vi "ArduinoRead.vi"(7 "Arduino function":enum16{"T/RH", "Interlock", "Edgesense"}(ring), 8 "error in (no error)":errorcluster, 9 "Humidity IN":dbl[](array[numeric]), 10 "Temperature IN":dbl[](array[numeric]), 11 "ArduinoControl in":refnum<class "ArduinoControl.lvclass">) -> (0 "error out":errorcluster, 1 "rel. Humidity [%]":dbl, 2 "Temperature [°C]":dbl, 3 "ArduinoControl out":refnum<class "ArduinoControl.lvclass">, 4 "Interlock Status":u16(ring) items=["Dark", "Light"], 5 "Edgesense Status":u16(ring)=1 items=["Contact", "No contact"])   [LabVIEW 2019, in "ArduinoControl.lvclass"]
uses:
  ArduinoControl.lvclass
  ArduinoControl.lvclass/ArduinoControl.ctl
panel:
  out "Humidity OUT":dbl[](array[numeric])
  out "Temperature OUT":dbl[](array[numeric])
  out "return count":u32
  out "String":string
  out "VISA resource name OUT":refnum<visa-resource-name>="COM24"
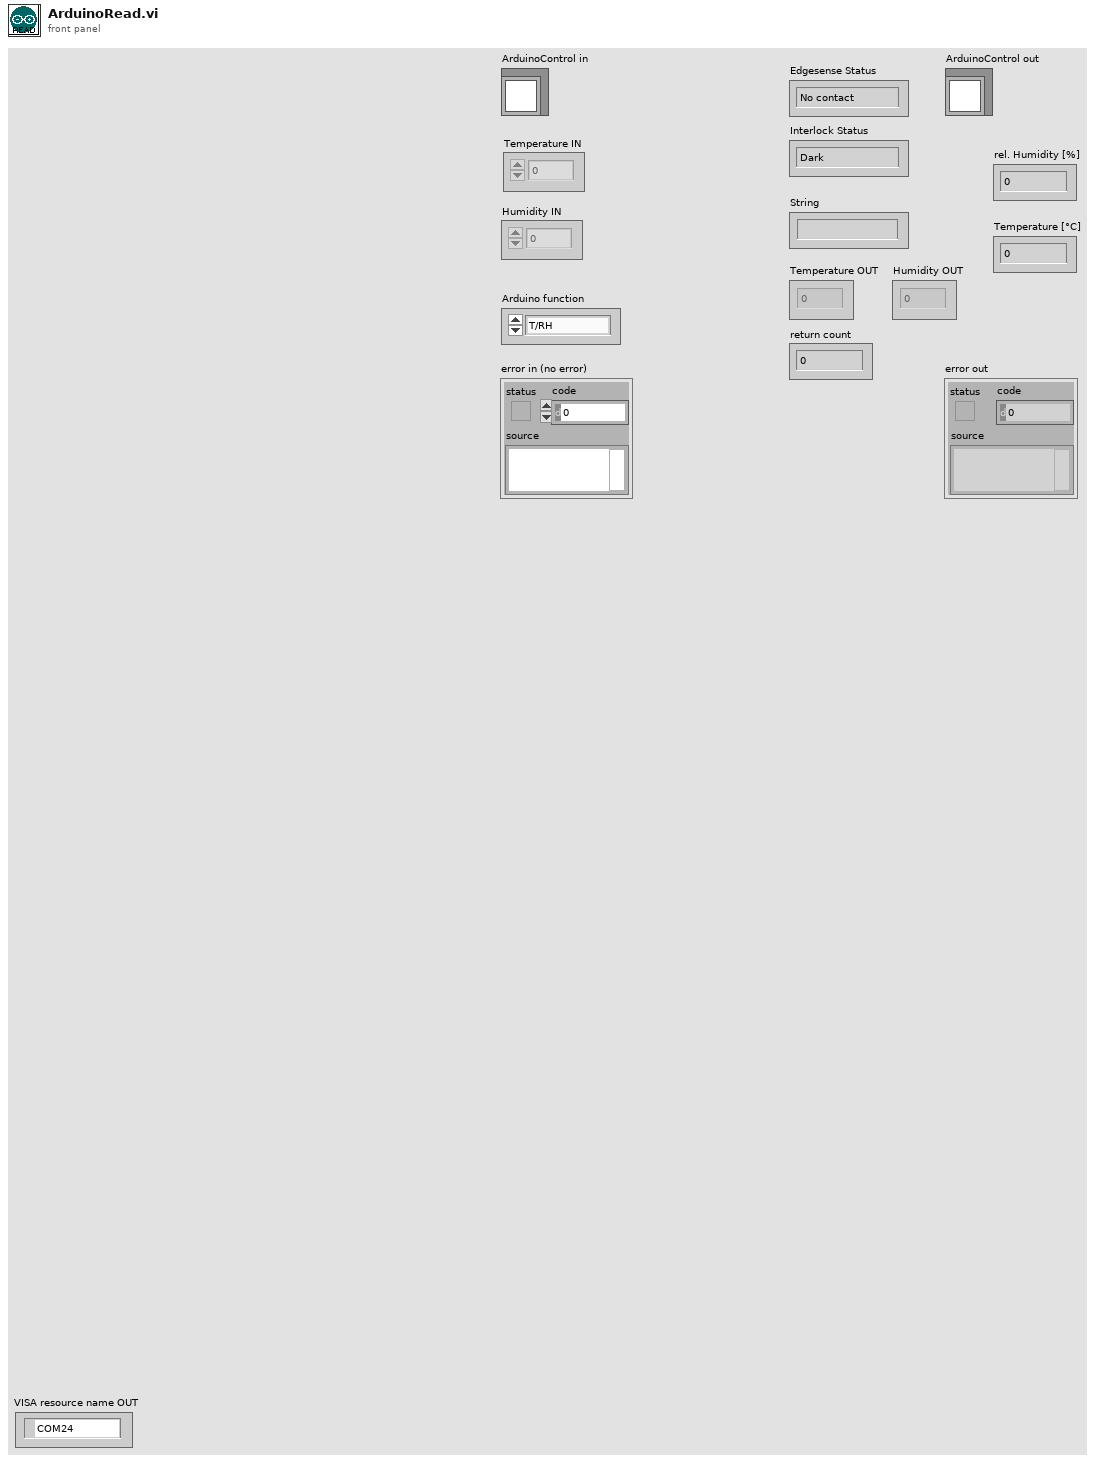
[diagram p1: front panel]
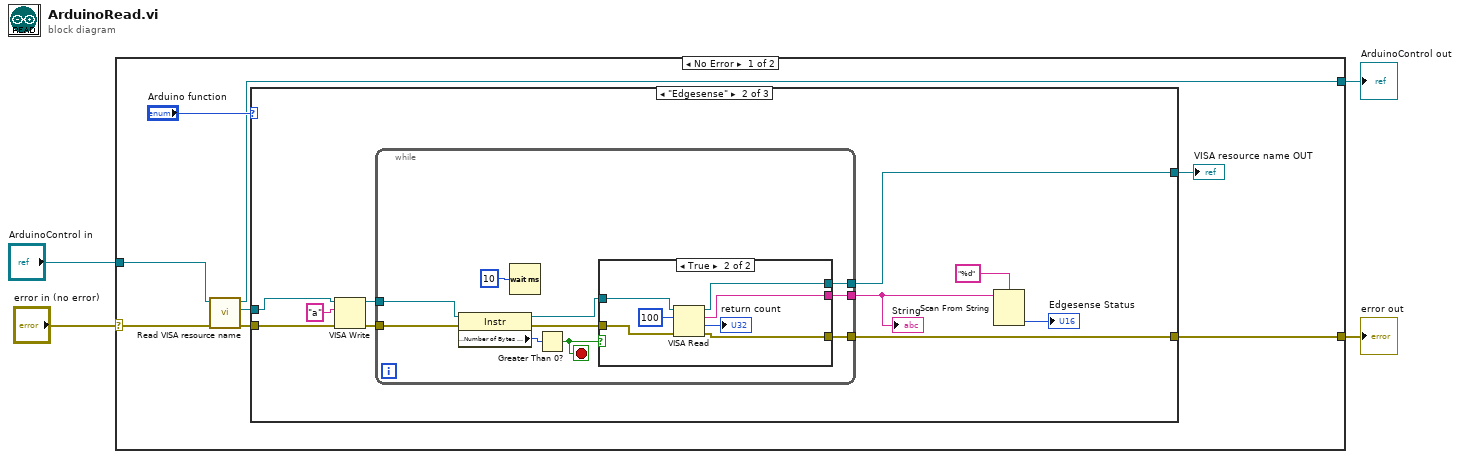
[diagram p0: block diagram]
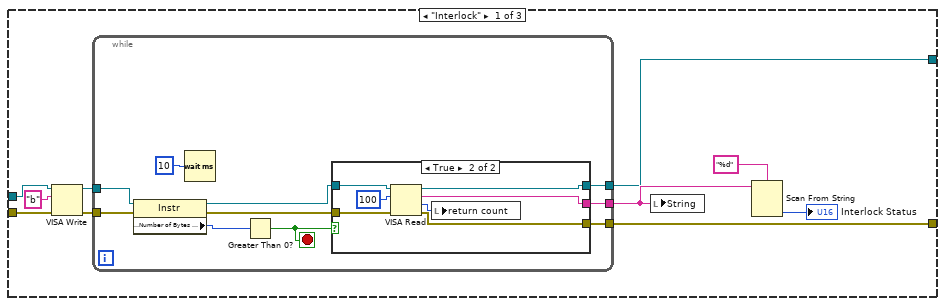
[diagram p2: hidden frame]
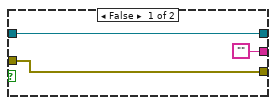
[diagram p3: hidden frame]
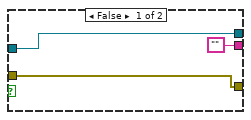
[diagram p4: hidden frame]
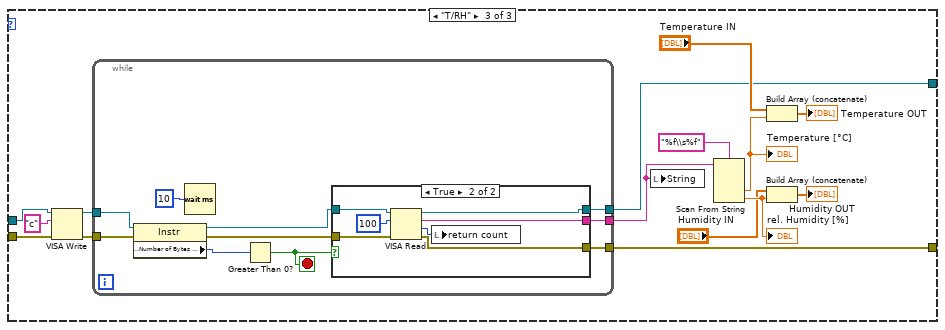
[diagram p5: hidden frame]
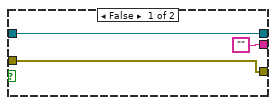
[diagram p6: hidden frame]
diagram:
  n1 = case shown="No Error" "error in (no error)" {
    selector: "error in (no error)" -> [w7 w109]
    tunnel: [w8 w108] -> w2
    tunnel: "ArduinoControl in" -> [w9 w108]
    tunnel: [w10 w109] -> w1
    frame No Error {
      n2 = call "Read VISA resource name.vi"("error in (no error)"=w7, "ArduinoControl in"=w9) -> ("error out"=w6:errorcluster, "VISA resource name"=w5:refnum<visa-resource-name>, "ArduinoControl out"=w8:refnum<class "ArduinoControl.lvclass">)  [unwired: 7 in]
      n3 = case shown="\"Edgesense\"" "Arduino function" {
        tunnel: w6 -> [w14 w45 w75]
        tunnel: w5 -> [w16 w46 w77]
        tunnel: [w19 w48 w78] -> w11
        tunnel: [w18 w49 w79] -> w10
        frame "Interlock" {
          n4 = VISA Write(VISA resource name=w16, write buffer="b", error in (no error)=w14) -> (VISA resource name out=w15:refnum<visa-resource-name>, error out=w13:errorcluster)  [unwired: 1 out]
          n5 = while {
            tunnel: [w30] -> w19
            tunnel: [w29] -> w20
            tunnel: w13 -> [w23]
            tunnel: w15 -> [w24]
            tunnel: [w28] -> w18
            stop <- w25 stop-if-true
            n6 = property class="Instr"(reference=w24, error in=w23) -> (reference out=w32:refnum<visa-resource-name>, error out=w31:errorcluster, "Serial Settings:Number of Bytes at Serial Port"=w26:u32)
            n7 = Wait (ms)(milliseconds to wait=10) -> ()  [unwired: 1 out]
            n8 = Greater Than 0?(x=w26) -> (x > 0?=w25:bool)
            n9 = case shown="True" w25 {
              tunnel: w32 -> [w33 w42]
              tunnel: w31 -> [w34 w41]
              tunnel: [w33 w40] -> w30
              tunnel: ["" w39] -> w29
              tunnel: [w34 w38] -> w28
              frame False {
              }
              frame True {
                n10 = VISA Read(VISA resource name=w42, byte count=100, error in (no error)=w41) -> (VISA resource name out=w40:refnum<visa-resource-name>, read buffer=w39:string, return count=w37:u32, error out=w38:errorcluster)
                n11 = local write "return count"(w37) -> ()
              }
            }
          }
          n12 = local write "String"(w20) -> ()
          n13 = Scan From String(format string="%d", input string=w20) -> (output 1=→"Interlock Status":u16)  [unwired: 3 in, 3 out]
        }
        frame "Edgesense" {
          n14 = VISA Write(VISA resource name=w46, write buffer="a", error in (no error)=w45) -> (VISA resource name out=w44:refnum<visa-resource-name>, error out=w43:errorcluster)  [unwired: 1 out]
          n15 = while {
            tunnel: [w60] -> w48
            tunnel: [w59] -> w50
            tunnel: w44 -> [w55]
            tunnel: [w58] -> w49
            tunnel: w43 -> [w56]
            stop <- w53 stop-if-true
            n16 = property class="Instr"(reference=w55, error in=w56) -> (reference out=w62:refnum<visa-resource-name>, error out=w61:errorcluster, "Serial Settings:Number of Bytes at Serial Port"=w54:u32)
            n17 = Wait (ms)(milliseconds to wait=10) -> ()  [unwired: 1 out]
            n18 = Greater Than 0?(x=w54) -> (x > 0?=w53:bool)
            n19 = case shown="True" w53 {
              tunnel: w62 -> [w63 w72]
              tunnel: w61 -> [w64 w71]
              tunnel: [w63 w70] -> w60
              tunnel: ["" w69] -> w59
              tunnel: [w64 w68] -> w58
              frame False {
              }
              frame True {
                n20 = VISA Read(VISA resource name=w72, byte count=100, error in (no error)=w71) -> (VISA resource name out=w70:refnum<visa-resource-name>, read buffer=w69:string, return count=→"return count":u32, error out=w68:errorcluster)
              }
            }
          }
          "String" <- w50
          n21 = Scan From String(format string="%d", input string=w50) -> (output 1=→"Edgesense Status":u16)  [unwired: 3 in, 3 out]
        }
        frame "T/RH" {
          n22 = VISA Write(VISA resource name=w77, write buffer="c", error in (no error)=w75) -> (VISA resource name out=w73:refnum<visa-resource-name>, error out=w74:errorcluster)  [unwired: 1 out]
          n23 = while {
            tunnel: [w95] -> w78
            tunnel: [w94] -> w80
            tunnel: w74 -> [w89]
            tunnel: w73 -> [w88]
            tunnel: [w93] -> w79
            stop <- w90 stop-if-true
            n24 = property class="Instr"(reference=w88, error in=w89) -> (reference out=w97:refnum<visa-resource-name>, error out=w96:errorcluster, "Serial Settings:Number of Bytes at Serial Port"=w91:u32)
            n25 = Wait (ms)(milliseconds to wait=10) -> ()  [unwired: 1 out]
            n26 = Greater Than 0?(x=w91) -> (x > 0?=w90:bool)
            n27 = case shown="True" w90 {
              tunnel: w97 -> [w98 w107]
              tunnel: w96 -> [w99 w106]
              tunnel: [w98 w105] -> w95
              tunnel: ["" w104] -> w94
              tunnel: [w99 w103] -> w93
              frame False {
              }
              frame True {
                n28 = VISA Read(VISA resource name=w107, byte count=100, error in (no error)=w106) -> (VISA resource name out=w105:refnum<visa-resource-name>, read buffer=w104:string, return count=w101:u32, error out=w103:errorcluster)
                n29 = local write "return count"(w101) -> ()
              }
            }
          }
          n30 = local write "String"(w80) -> ()
          n31 = Scan From String(format string="%f\\s%f", input string=w80) -> (output 1=w82:dbl, output 2=w87:dbl)  [unwired: 4 in, 3 out]
          "rel. Humidity [%]" <- w87
          "Temperature [°C]" <- w82
          n32 = Build Array (concatenate)("Temperature IN", w82) -> (→"Temperature OUT":dbl[])
          n33 = Build Array (concatenate)("Humidity IN", w87) -> (→"Humidity OUT":dbl[])
        }
      }
      "VISA resource name OUT" <- w11
    }
    frame Error {
    }
  }
  "error out" <- w1
  "ArduinoControl out" <- w2
